vi "CMI ADS127L21 - Open.vi"(8 "error in (no error)":errorcluster, 11 "session in":T1 {"channels"."Channel" min=1 max=8 step=1; "channels"."Range [Vpk]" items=["±1.65V", "±2V"]}) -> (0 "error out":errorcluster, 2 "idn string":string, 3 "session out":T1 {"channels"."Channel" min=1 max=8 step=1; "channels"."Range [Vpk]" items=["±1.65V", "±2V"]})   [LabVIEW 2020]
doc: "Open digitizer."
uses:
  CMI ADS127L21 - Session.ctl
  CMI ADS127L21 - Record Channel.ctl
  CMI ADS127L21 - Input Range.ctl
  CMI ADS127L21 - Input Mode.ctl
  CMI ADS127L21 - Input Impedance.ctl
  CMI ADS127L21 - EXTOUT Mode.ctl
  CMI ADS127L21 - EXTOUT Polarity.ctl
  <vilib>/Instr/_visa.llb/VISA Flush IO Buffer Mask.ctl
  <vilib>/Utility/error.llb/Error Cluster From Error Code.vi
  <vilib>/ErrorRing/Error Ring.xnode
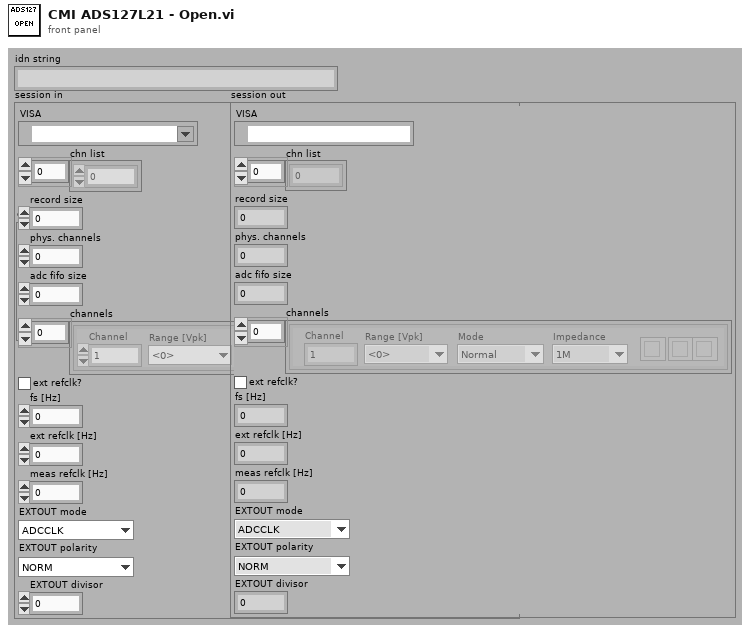
[diagram p1: front panel]
types:
  T1 = typedef "CMI ADS127L21 - Session.ctl" = cluster{"VISA":refnum<visa-resource-name>, "chn list":i32[], "record size":i32, "phys. channels":i32, "adc fifo size":i32, "channels":T2[], "ext refclk?":bool, "fs [Hz]":dbl, "ext refclk [Hz]":dbl, "meas refclk [Hz]":dbl, "EXTOUT mode":T6, "EXTOUT polarity":T7, "EXTOUT divisor":i32}
  T2 = typedef "CMI ADS127L21 - Record Channel.ctl" = cluster{"Range [Vpk]":T3, "Channel":i32, "Mode":T4, "Impedance":T5, "btn clr":bool, "btn up":bool, "btn down":bool}
  T3 = typedef "CMI ADS127L21 - Input Range.ctl" = dbl
  T4 = typedef "CMI ADS127L21 - Input Mode.ctl" = enum16{"Normal", "Inverted", "GND"}
  T5 = typedef "CMI ADS127L21 - Input Impedance.ctl" = enum16{"1M", "1k5"}
  T6 = typedef "CMI ADS127L21 - EXTOUT Mode.ctl" = enum16{"ADCCLK", "REFCLK", "SMPLCLK", "FIRST"}
  T7 = typedef "CMI ADS127L21 - EXTOUT Polarity.ctl" = enum16{"NORM", "INV"}
  T8 = typedef "VISA Flush IO Buffer Mask.ctl" = u16
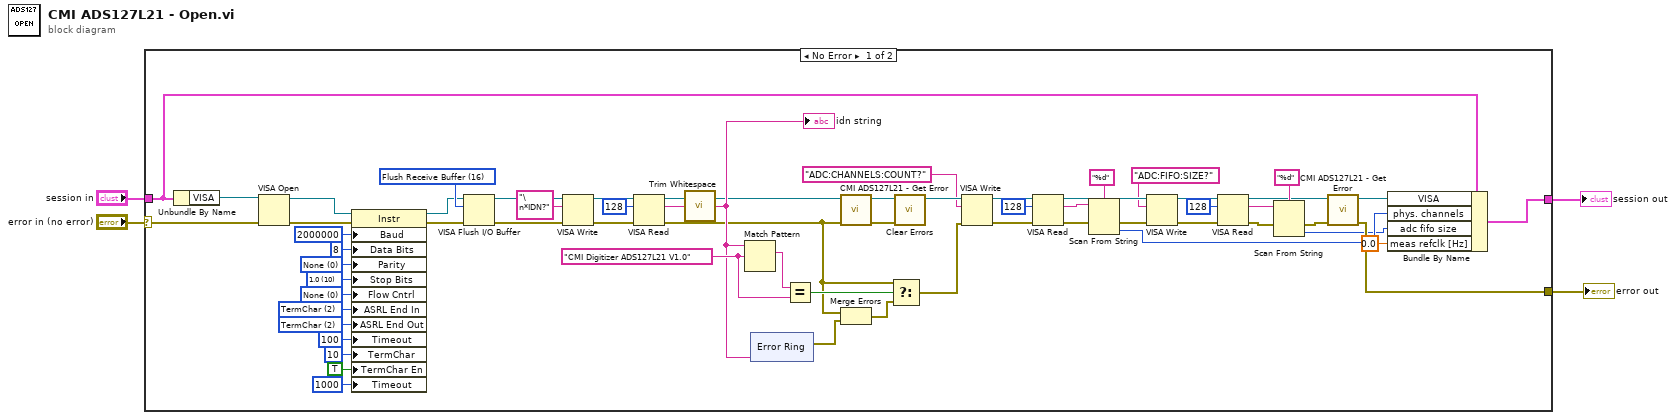
[diagram p0: block diagram]
diagram:
  n1 = case shown="No Error" "error in (no error)" {
    selector: "error in (no error)" -> [w31 w73]
    tunnel: [w9 w73] -> w4
    tunnel: [w33 w74] -> w3
    tunnel: "session in" -> [w32 w74]
    frame No Error {
      w43 = "CMI Digitizer ADS127L21 V1.0" ("regular expression")
      w55 = u16 2 items=["None", "Last Bit", "TermChar", "Break"] ("Serial Settings:End Mode for Writes")
      w56 = u16 2 items=["None", "Last Bit", "TermChar"] ("Serial Settings:End Mode for Reads")
      w57 = u16 0 items=["None", "XON/XOFF", "RTS/CTS", "XON/XOFF & RTS/CTS", "DTR/DSR", "XON/XOFF & DTR/DSR"] ("Serial Settings:Flow Control")
      w58 = u16 10 items=["1.0"=10, "1.5"=15, "2.0"=20] ("Serial Settings:Stop Bits")
      w59 = u16 0 items=["None", "Odd", "Even", "Mark", "Space"] ("Serial Settings:Parity")
      w65 = T8 16 items=["Flush Receive Buffer"=16, "Write Transmit Buffer to Device"=32, "Flush Receive Buffer (No I/O)"=64, "Flush Transmit Buffer"=128] ("Mask")
      n2 = Unbundle By Name(w32) -> ("VISA"=w34:refnum<visa-resource-name>)
      n3 = VISA Open(error in (no error)=w31, VISA resource name=w34) -> (VISA resource name=w63:refnum<visa-resource-name>, error out=w64:errorcluster)  [unwired: 3 in]
      n4 = property class="Instr"(reference=w63, error in=w64, "Baud"=u32 2000000 ("Serial Settings:Baud Rate"), "Data Bits"=u16 8 ("Serial Settings:Data Bits"), "Parity"=w59, "Stop Bits"=w58, "Flow Cntrl"=w57, "ASRL End In"=w56, "ASRL End Out"=w55, "Timeout"=u32 100 ("General Settings:Timeout Value"), "TermChar"=u8 10 ("Message Based Settings:Termination Character"), "TermChar En"=TRUE ("Message Based Settings:Termination Character Enable"), "Timeout"=u32 1000 ("General Settings:Timeout Value")) -> (reference out=w62:refnum<visa-resource-name>, error out=w51:errorcluster)
      n5 = VISA Flush I/O Buffer(VISA resource name=w62, mask (16)=w65, error in (no error)=w51) -> (VISA resource name out=w49:refnum<visa-resource-name>, error out=w50:errorcluster)
      n6 = VISA Write(VISA resource name=w49, write buffer="\n*IDN?", error in (no error)=w50) -> (VISA resource name out=w46:refnum<visa-resource-name>, error out=w47:errorcluster)  [unwired: 1 out]
      n7 = VISA Read(VISA resource name=w46, byte count=u32 128, error in (no error)=w47) -> (VISA resource name out=w36:refnum<visa-resource-name>, read buffer=w39:string, error out=w37:errorcluster)  [unwired: 1 out]
      n8 = call <vilib>:"Trim Whitespace.vi"("string"=w39) -> ("trimmed string"=w38:string)  [unwired: 1 in]
      "idn string" <- w38
      n9 = Match Pattern(string=w38, regular expression=w43) -> (match substring=w44:string)  [unwired: 1 in, 3 out]
      n10 = xnode "Error Ring"("parameter 0"=w38) -> ("error out"=w40:errorcluster)
      n11 = Equal?(x=w44, y=w43) -> (x = y?=w42:bool)
      n12 = call "CMI ADS127L21 - Get Error.vi"("error in (no error)"=w37, "VISA in"=w36) -> ("error out"=w35:errorcluster, "VISA out"=w27:refnum<visa-resource-name>)  [unwired: 8 in]
      n13 = Merge Errors(w37, w40) -> (w41:errorcluster)
      n14 = Select(t=w37, s=w42, f=w41) -> (s? t:f=w13:errorcluster)
      n15 = call <vilib>:"Clear Errors.vi"("error in (no error)"=w35) -> ()  [unwired: 5 in, 2 out]
      n16 = VISA Write(VISA resource name=w27, write buffer="ADC:CHANNELS:COUNT?", error in (no error)=w13) -> (VISA resource name out=w29:refnum<visa-resource-name>, error out=w28:errorcluster)  [unwired: 1 out]
      n17 = VISA Read(VISA resource name=w29, byte count=u32 128, error in (no error)=w28) -> (VISA resource name out=w15:refnum<visa-resource-name>, read buffer=w24:string, error out=w25:errorcluster)  [unwired: 1 out]
      n18 = Scan From String(format string="%d", input string=w24, error in=w25) -> (error out=w16:errorcluster, output 1=w8:i32)  [unwired: 2 in, 2 out]
      n19 = VISA Write(VISA resource name=w15, write buffer="ADC:FIFO:SIZE?", error in (no error)=w16) -> (VISA resource name out=w18:refnum<visa-resource-name>, error out=w19:errorcluster)  [unwired: 1 out]
      n20 = VISA Read(VISA resource name=w18, byte count=u32 128, error in (no error)=w19) -> (VISA resource name out=w11:refnum<visa-resource-name>, read buffer=w21:string, error out=w20:errorcluster)  [unwired: 1 out]
      n21 = Scan From String(format string="%d", input string=w21, error in=w20) -> (error out=w12:errorcluster, output 1=w7:i32)  [unwired: 2 in, 2 out]
      n22 = call "CMI ADS127L21 - Get Error.vi"("error in (no error)"=w12, "VISA in"=w11) -> ("error out"=w9:errorcluster, "VISA out"=w10:refnum<visa-resource-name>)  [unwired: 8 in]
      n23 = Bundle By Name(cluster=w32, "VISA"=w10, "phys. channels"=w8, "adc fifo size"=w7, "meas refclk [Hz]"=0.0) -> (w33:T1)
    }
    frame Error {
    }
  }
  "error out" <- w4
  "session out" <- w3
